vi "CSM - MassData Update Status Indicator.vi"(8 "error in (no error)":errorcluster, 11 "MassData Status Indicator":refnum<vi>) -> (0 "error out":errorcluster)   [LabVIEW 2017]
doc: "Helper VI to update the specified Massdata cache display control on the UI based on the cache status, allowing for a more intuitive visualization of cache usage.\n\n-- <b>Controls</b> --\n- <b>MassData Status Indicator</b>: Reference to the Massdata cache display control."
uses:
  Def-MassData Status Indicator(Vertical).ctl
  _support/Operation-FGV-MassData.ctl
  CSM MassData Parameter Support.lvlib
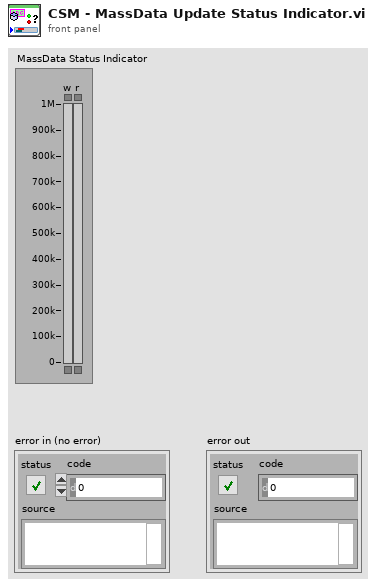
[diagram p1: front panel]
types:
  T1 = typedef "CSM MassData Parameter Support.lvlib/Operation-FGV-MassData.ctl" = enum16{"Initialize", "Read", "Write", "Status", "Release"}
  T2 = typedef "CSM MassData Parameter Support.lvlib/Def-MassDataOper-Status.ctl" = cluster{"Start":i32, "Size":i32, "Total":i32}
  T3 = cluster{cluster{i32, "Start":i32}, cluster{i32, "Start":i32}}
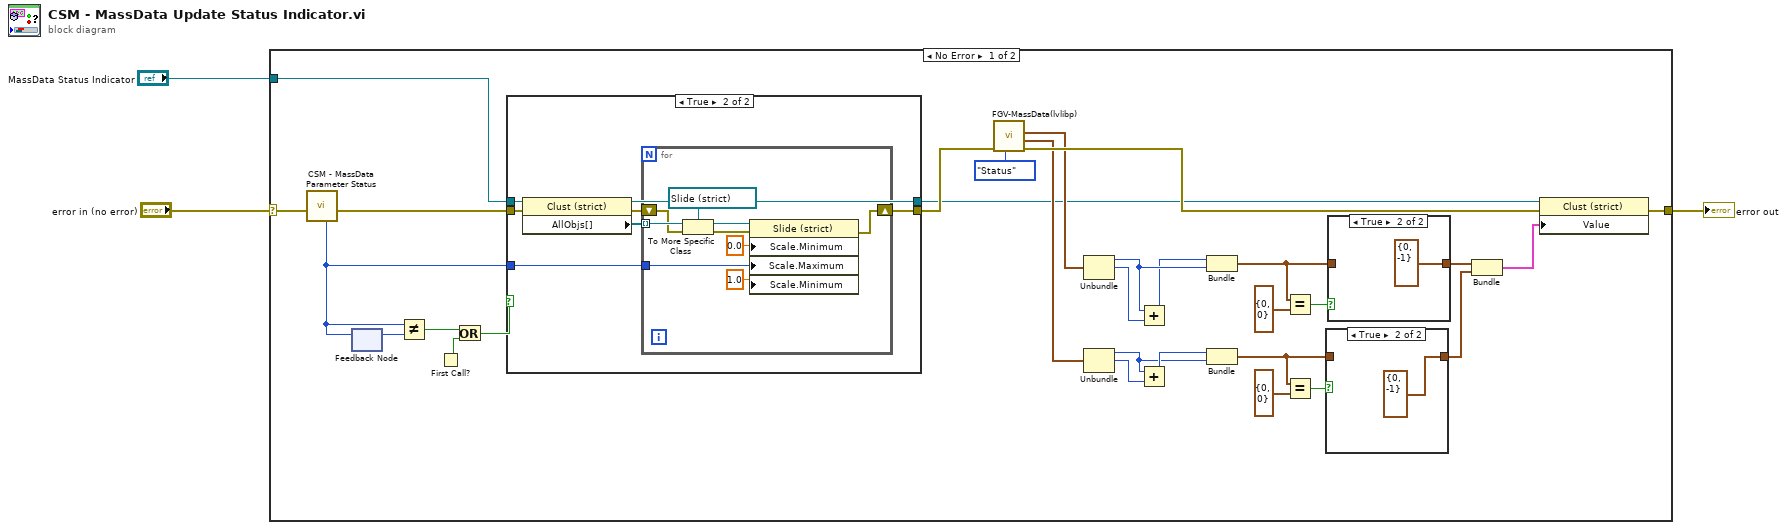
[diagram p0: block diagram]
diagram:
  n1 = case shown="No Error" "error in (no error)" {
    selector: "error in (no error)" -> [w21 w56]
    tunnel: [w33 w56] -> w3
    tunnel: "MassData Status Indicator" -> [w17 _]
    frame No Error {
      n2 = call "CSM - MassData Parameter Status.vi"("Error in"=w21) -> ("Error out"=w20:errorcluster, "Cache Size"=w14:i32)  [unwired: 6 in, 2 out]
      n3 = feedback-in #1(w14) -> ()
      n4 = feedback #1() -> (w13:i32)  [unwired: 1 in]
      n5 = Not Equal?(x=w14, y=w13) -> (x != y?=w12:bool)
      n6 = First Call?() -> (First Call?: T/F=w18:bool)
      n7 = Or(x=w12, y=w18) -> (x .or. y?=w15:bool)
      n8 = case shown="True" w15 {
        tunnel: w20 -> [w39 w46]
        tunnel: [w39 w43] -> w19
        tunnel: w14 -> [_ w42]
        tunnel: w17 -> [w38 w41]
        tunnel: [w38 w40] -> w16
        frame False {
        }
        frame True {
          n9 = property on="Property Node" class="Clust (strict)"(reference=w41, error in=w46) -> (reference out=w40:refnum<vi>, error out=w44:errorcluster, "AllObjs[]"=w45:refnum<vi>[])
          n10 = for {
            tunnel: w45 -> [w55] mode=indexing
            tunnel: w42 -> [w52]
            shift-right: [w47] -> w43
            shift-left: w44 -> [w49]
            n11 = To More Specific Class(target class=refnum<vi> refnum ("w"), reference=w55, error in=w49) -> (specific class reference=w54:refnum<vi>, error out=w48:errorcluster)
            n12 = property on="Property Node" class="Slide (strict)"(reference=w54, error in=w48, "Scale.Minimum"=0.0 ("Scale.Range:Minimum"), "Scale.Maximum"=w52, "Scale.Minimum"=1.0 ("Scale.Range:Minimum")) -> (error out=w47:errorcluster)  [unwired: 1 out]
          }
        }
      }
      n13 = call "FGV-MassData(lvlibp).vi"("Operation"=Operation-FGV-MassData."Status", "Error in"=w19) -> ("Error out"=w31:errorcluster, "Active Read Oper"=w22:T2, "Active Write Oper"=w26:T2)  [unwired: 6 in, 1 out]
      n14 = Unbundle(w26) -> ("Start"=w29:i32, "Size"=w27:i32)  [unwired: 1 out]
      n15 = Unbundle(w22) -> ("Start"=w23:i32, "Size"=w25:i32)  [unwired: 1 out]
      n16 = Add(x=w29, y=w27) -> (x+y=w28:i32)
      n17 = Add(x=w23, y=w25) -> (x+y=w24:i32)
      n18 = Bundle(w28, "Start"=w29) -> (w5:cluster{i32, "Start":i32})  [unwired: 1 in]
      n19 = Bundle(w24, "Start"=w23) -> (w7:cluster{i32, "Start":i32})  [unwired: 1 in]
      n20 = Equal?(x=w5, y=cluster{i32, "Start":i32} {0, "Start"=0}) -> (x = y?=w10:bool)
      n21 = Equal?(x=w7, y=cluster{i32, "Start":i32} {0, "Start"=0}) -> (x = y?=w8:bool)
      n22 = case shown="True" w8 {
        tunnel: w7 -> [w34 _]
        tunnel: [w34 cluster{i32, "Start":i32} {0, "Start"=-1}] -> w4
        frame False {
        }
        frame True {
        }
      }
      n23 = case shown="True" w10 {
        tunnel: [w36 cluster{i32, "Start":i32} {0, "Start"=-1}] -> w6
        tunnel: w5 -> [w36 _]
        frame False {
        }
        frame True {
        }
      }
      n24 = Bundle(w6, w4) -> (w32:T3)  [unwired: 1 in]
      n25 = property on="Property Node" class="Clust (strict)"(reference=w16, error in=w31, "Value"=w32) -> (error out=w33:errorcluster)  [unwired: 1 out]
    }
    frame Error {
    }
  }
  "error out" <- w3
